vi "Timer.vi"(7 "CMD":enum16{"Reset", "Check"}(ring), 8 "error in (no error)":errorcluster, 10 "Time Stamp":timestamp) -> (0 "error out":errorcluster, 2 "Elapsed (minutes)":dbl, 3 "Elapsed (seconds)":dbl)   [LabVIEW 2017]
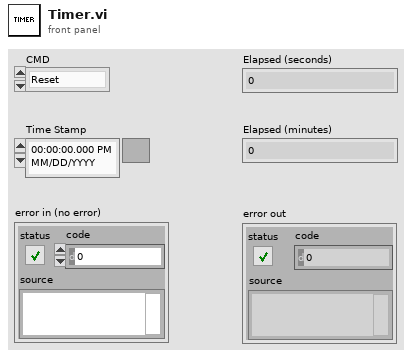
[diagram p1: front panel]
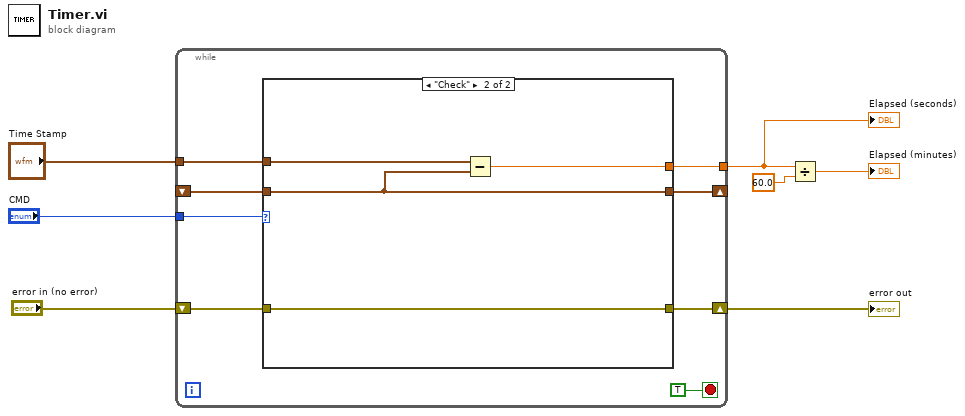
[diagram p0: block diagram]
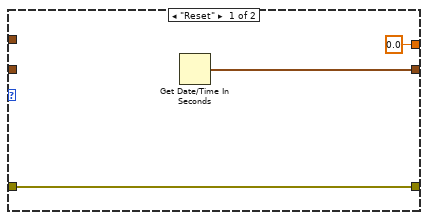
[diagram p2: hidden frame]
diagram:
  n1 = while {
    shift-right: [w13] -> w6
    shift-left: "error in (no error)" -> [w14]
    tunnel: "CMD" -> [w12]
    tunnel: "Time Stamp" -> [w11]
    shift-right: [w10] -> _
    shift-left: _ -> [w9]
    tunnel: [w8] -> w1
    stop <- TRUE stop-if-true
    n2 = case shown="\"Check\"" w12 {
      tunnel: w14 -> [w18 w22]
      tunnel: [w18 w22] -> w13
      tunnel: w11 -> [_ w21]
      tunnel: [w17 w20] -> w10
      tunnel: w9 -> [_ w20]
      tunnel: [0.0 w19] -> w8
      frame "Reset" {
        n3 = Get Date/Time In Seconds() -> (seconds since 1Jan1904=w17:timestamp)
      }
      frame "Check" {
        n4 = Subtract(x=w21, y=w20) -> (x-y=w19:dbl)
      }
    }
  }
  "error out" <- w6
  "Elapsed (seconds)" <- w1
  n5 = Divide(x=w1, y=60.0 ("x")) -> (x/y=→"Elapsed (minutes)":dbl)
